vi "ep_Reference Channel Process.vi"(7 "reset? (F)":bool, 8 "error in (no error)":errorcluster, 9 "system info in":refnum<class "EP System Info.lvclass">, 10 "dt":dbl, 11 "reference data":dbl[](array[numeric])) -> (0 "error out":errorcluster, 1 "system info out":refnum<class "EP System Info.lvclass">, 2 "time position":dbl[](array[numeric]), 3 "sampling rate [Hz]":dbl)   [LabVIEW 2013, in "NI_EP_Resample_Host.lvlib"]
uses:
  <vilib>/addons/Electrical Power/PQ/Resampling/NI_EP_Resample_Host.lvlib
  <vilib>/addons/Electrical Power/PQ/Common/Classes/System Info/EP System Info.lvclass
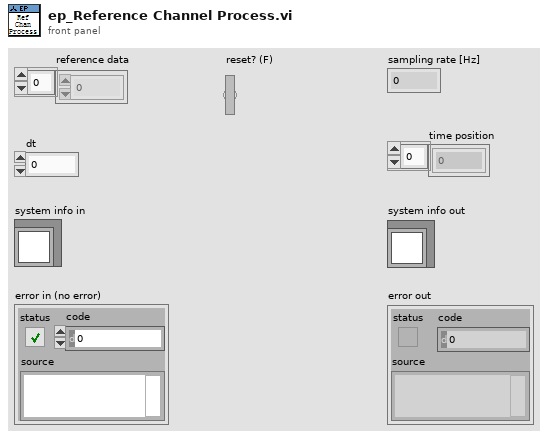
[diagram p1: front panel]
types:
  T1 = typedef "NI_EP_Resample_Host.lvlib/ep_Parameters.ctl" = cluster{"filter parameters":cluster{"enable filter":bool, "lp filter coefficients":dbl[], "bp filter coefficients":dbl[]}, "fs after decimation":dbl, "decimation factor":i32, "norminal frequency":dbl, "norminal hf prd samp":dbl, "lower hf prd samp":i32, "upper hf prd samp":i32}
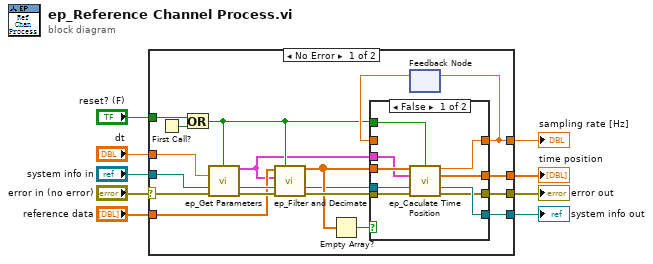
[diagram p0: block diagram]
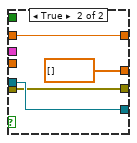
[diagram p2: hidden frame]
diagram:
  n1 = case shown="No Error" "error in (no error)" {
    selector: "error in (no error)" -> [w20 w41]
    tunnel: "system info in" -> [w21 w42]
    tunnel: [w18 w42] -> w8
    tunnel: [w17 w41] -> w7
    tunnel: "reset? (F)" -> [w26 _]
    tunnel: "dt" -> [w15 _]
    tunnel: "reference data" -> [w11 _]
    tunnel: [w14 _] -> w2
    tunnel: [w13 _] -> w1
    frame No Error {
      n2 = First Call?() -> (First Call?: T/F=w27:bool)
      n3 = Or(x=w26, y=w27) -> (x .or. y?=w16:bool)
      n4 = call <vilib>:"ep_Get Parameters.vi"("reset? (F)"=w16, "dt"=w15, "system info in"=w21, "error in (no error)"=w20) -> ("parameters"=w10:T1, "system info out"=w12:refnum<class "EP System Info.lvclass">, "error out"=w19:errorcluster)  [unwired: 9 in]
      n5 = call <vilib>:"ep_Filter and Decimate.vi"("reset? (F)"=w16, "error in (no error)"=w19, "parameters"=w10, "data in"=w11) -> ("error out"=w25:errorcluster, "data out"=w23:dbl[])  [unwired: 5 in, 1 out]
      n6 = Empty Array?(array=w23) -> (empty?=w24:bool)
      n7 = feedback #1() -> (w22:dbl)  [unwired: 1 in]
      n8 = case shown="False" w24 {
        tunnel: w25 -> [w36 w39]
        tunnel: w12 -> [w35 w40]
        tunnel: w23 -> [w34 _]
        tunnel: [w33 dbl[] [] ("time position")] -> w14
        tunnel: w16 -> [w28 _]
        tunnel: [w32 w40] -> w18
        tunnel: [w31 w38] -> w13
        tunnel: [w30 w39] -> w17
        tunnel: w22 -> [_ w38]
        tunnel: w10 -> [w29 _]
        frame False {
          n9 = call <vilib>:"ep_Caculate Time Position.vi"("reference signal"=w34, "reset? (F)"=w28, "parameters"=w29, "system info in"=w35, "error in (no error)"=w36) -> ("sampling rate [Hz]"=w31:dbl, "time position"=w33:dbl[], "system info out"=w32:refnum<class "EP System Info.lvclass">, "error out"=w30:errorcluster)  [unwired: 7 in]
        }
        frame True {
        }
      }
      n10 = feedback-in #1(w13) -> ()
    }
    frame Error {
    }
  }
  "error out" <- w7
  "system info out" <- w8
  "time position" <- w2
  "sampling rate [Hz]" <- w1
